vi "Interpolation Settings.vi"(6 "Action":T2, 8 "error in (no error)":errorcluster, 10 "Interpolation Settings":T1, 11 "Item Ref":T3 format="%.0x") -> (0 "error out":errorcluster, 2 "Interpolation Settings out":T1, 3 "Item Ref out":T3=18446744073709551615 format="%.0x")   [LabVIEW 2019, in "Profile Interpolation Shared.lvlib"]
uses:
  Profile Interpolation Shared.lvlib
  <vilib>/NI VeriStand/Custom Device API/Custom Device Item Ref.ctl
  Types/FG Action.ctl
  Types/Interpolation Settings.ctl
  Constants.vi
  <vilib>/NI VeriStand/Custom Device API/Get Item Property (Path).vi
  <vilib>/NI VeriStand/Custom Device API/Get Item Property (Boolean).vi
  <vilib>/NI VeriStand/Custom Device API/Set Item Property (Path).vi
  <vilib>/NI VeriStand/Custom Device API/Set Item Property (Boolean).vi
  <vilib>/NI VeriStand/Custom Device API/Custom Device API.lvlib
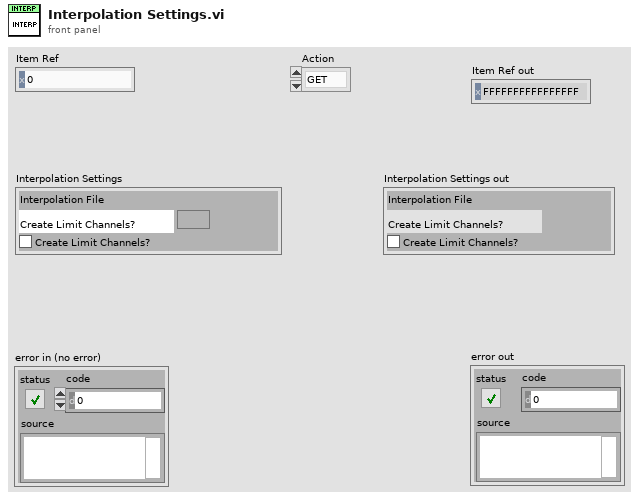
[diagram p1: front panel]
types:
  T1 = typedef "Profile Interpolation Shared.lvlib/Interpolation Settings.ctl" = cluster{"Interpolation File":path, "Create Limit Channels?":bool}
  T2 = typedef "Profile Interpolation Shared.lvlib/FG Action.ctl" = enum8{"GET", "SET"}
  T3 = typedef "Custom Device API.lvlib/Custom Device Item Ref.ctl" = u64
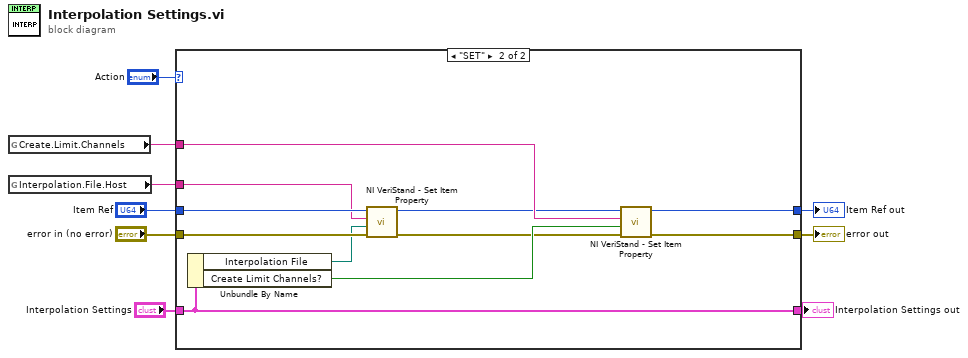
[diagram p0: block diagram]
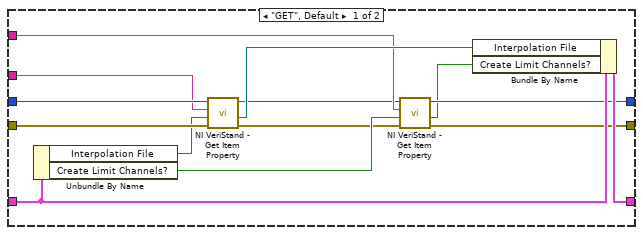
[diagram p2: hidden frame]
diagram:
  n1 = global read "Constants.vi" "Create.Limit.Channels"() -> (w1:string)
  n2 = global read "Constants.vi" "Interpolation.File.Host"() -> (w4:string)
  n3 = case shown="\"SET\"" "Action" {
    tunnel: "error in (no error)" -> [w23 w34]
    tunnel: "Item Ref" -> [w22 w33]
    tunnel: "Interpolation Settings" -> [w20 w32]
    tunnel: [w16 w29] -> w9
    tunnel: [w15 w26] -> w6
    tunnel: [w19 w32] -> w2
    tunnel: w4 -> [w18 w31]
    tunnel: w1 -> [w12 w27]
    frame "GET", Default {
      n4 = Unbundle By Name(w20) -> ("Interpolation File"=w21:path, "Create Limit Channels?"=w13:bool)
      n5 = call-poly <vilib>:"NI VeriStand - Get Item Property.vi"("error in (no error)"=w23, "Default Value"=w21, "Property Name"=w18, "Item Ref in"=w22) -> ("error out"=w10:errorcluster, "Value"=w17:path, "Item Ref out"=w11:T3)  [unwired: 4 in, 1 out]
      n6 = call-poly <vilib>:"NI VeriStand - Get Item Property.vi"("error in (no error)"=w10, "Default Value"=w13, "Property Name"=w12, "Item Ref in"=w11) -> ("error out"=w16:errorcluster, "Value"=w14:bool, "Item Ref out"=w15:T3)  [unwired: 4 in, 1 out]
      n7 = Bundle By Name(cluster=w20, "Interpolation File"=w17, "Create Limit Channels?"=w14) -> (w19:T1)
    }
    frame "SET" {
      n8 = Unbundle By Name(w32) -> ("Interpolation File"=w30:path, "Create Limit Channels?"=w28:bool)
      n9 = call-poly <vilib>:"NI VeriStand - Set Item Property.vi"("error in (no error)"=w34, "Value"=w30, "Property Name"=w31, "Item Ref in"=w33) -> ("error out"=w24:errorcluster, "Item Ref out"=w25:T3)  [unwired: 5 in, 1 out]
      n10 = call-poly <vilib>:"NI VeriStand - Set Item Property.vi"("error in (no error)"=w24, "Value"=w28, "Property Name"=w27, "Item Ref in"=w25) -> ("error out"=w29:errorcluster, "Item Ref out"=w26:T3)  [unwired: 5 in, 1 out]
    }
  }
  "error out" <- w9
  "Item Ref out" <- w6
  "Interpolation Settings out" <- w2
